vi "K237-read-current-2.vi"(2 "error in":T1, 3 "GPIB":string) -> (0 "error out":T1, 1 "Current":dbl)   [LabVIEW 2009]
panel:
  out "status":bool[](array[boolean])
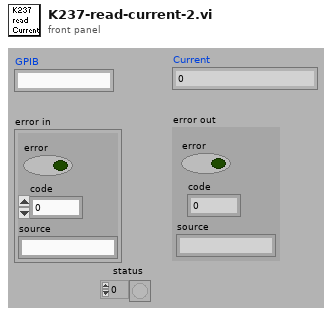
[diagram p1: front panel]
types:
  T1 = cluster{"error":bool, "code":i32, "source":string}
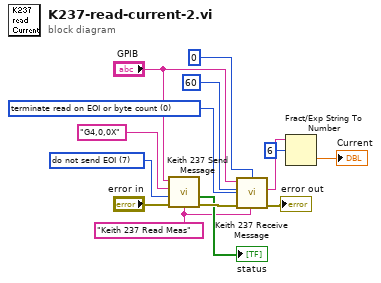
[diagram p0: block diagram]
diagram:
  w2 = "Keith 237 Read Meas" ("source")
  w4 = 0 items=["terminate read on EOI or byte count", "terminate read on EOI, byte count, or CR", "terminate read on EOI, byte count, or LF"] ("read mode (EOI:0)")
  w5 = 7 items=["send EOI with last character of string", "append CR to string and send EOI with CR", "append LF to string and send EOI with LF", "append CR LF to string and send EOI with LF", "append CR to string but do not send EOI", "append LF to string but do not send EOI", "append CR LF to string but do not send EOI", "do not send EOI"] ("write mode (send EOI:0)")
  n1 = call "Keith 237 Send Message.vi"("address string"="GPIB", "write buffer"="G4,0,0X", "source"=w2, "write mode (send EOI:0)"=w5, "error in"="error in") -> ("status"=→"status":bool[], "error out"=w10:T1)  [unwired: 1 in, 2 out]
  n2 = call <instrlib>:"Keith 237 Receive Message.vi"("timeout ms"=u32 0, "address string"="GPIB", "byte count"=60, "source"=w2, "read mode (EOI:0)"=w4, "error in"=w10) -> ("read buffer"=w3:string, "error out"=→"error out":T1)  [unwired: 2 out]
  n3 = Fract/Exp String To Number(string=w3, offset=6) -> (number=→"Current":dbl)  [unwired: 3 out]
